vi "bind text.vi"(8 "error in (no error)":errorcluster, 10 "String":string, 11 "SQLite3LV Cursor in":refnum<class "cursor.lvclass">) -> (0 "error out":errorcluster, 3 "SQLite3LV Cursor out":refnum<class "cursor.lvclass">)   [LabVIEW 2014, in "SQLite3LV.lvlib" / "cursor.lvclass"]
uses:
  cursor.lvclass
  cursor.lvclass/cursor.ctl
  SQLite3LV.lvlib
  sqlite3_64.dll
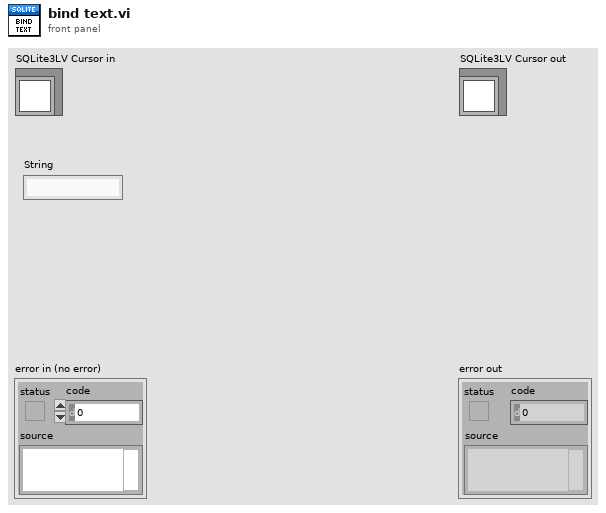
[diagram p1: front panel]
types:
  T1 = typedef "SQLite3LV.lvlib/cursor.lvclass/ctl_active_statement.ctl" = cluster{"ppStmt":i64, "column count":i32, "bind offset":i32, "bind param count":i32, "finished?":bool, "column offset":i32, "column types":i32[]}
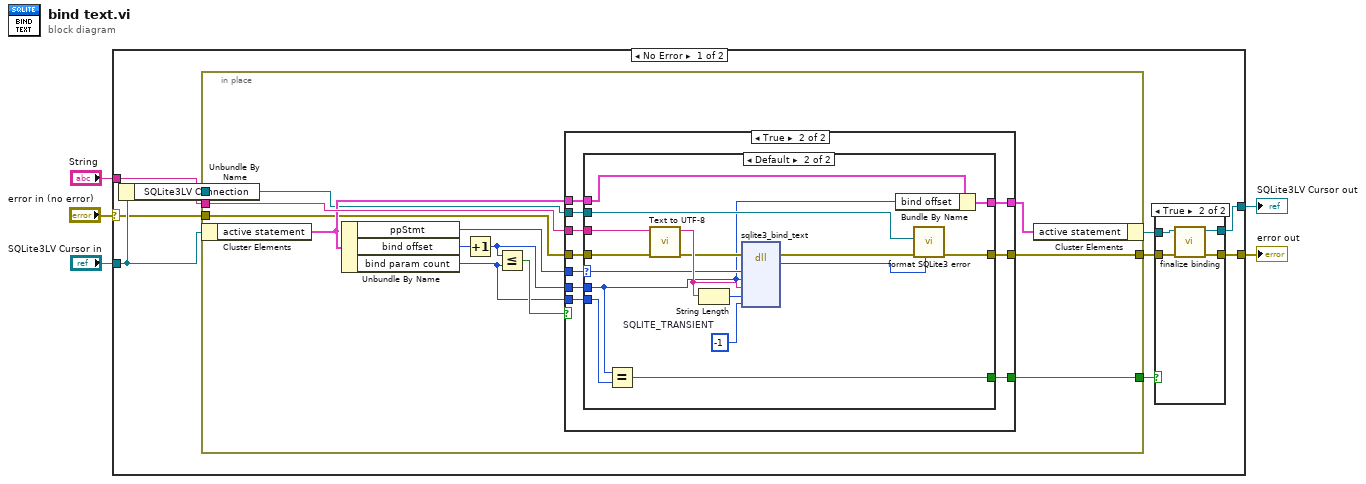
[diagram p0: block diagram]
diagram:
  n1 = case shown="No Error" "error in (no error)" {
    selector: "error in (no error)" -> [w7 w63]
    tunnel: [w10 w63] -> w4
    tunnel: [w12 w62] -> w3
    tunnel: "SQLite3LV Cursor in" -> [w9 w62]
    tunnel: "String" -> [w14 _]
    frame No Error {
      n2 = Unbundle By Name(w9) -> ("SQLite3LV Connection"=w8:refnum<class "sqlite3.lvclass">)
      n3 = in-place {
        in-place-border: w14 -> [w32]
        in-place-border: [w31] -> w11
        in-place-border: w8 -> [w24]
        in-place-border: w7 -> [w23]
        in-place-border: [w21] -> w6
        n4 = in-place-cluster #1(w9) -> ("active statement"=w26:T1)
        n5 = Unbundle By Name(w26) -> ("ppStmt"=w30:i64, "bind offset"=w29:i32, "bind param count"=w22:i32)
        n6 = Increment(x=w29) -> (x+1=w28:i32)
        n7 = Less Or Equal?(x=w28, y=w22) -> (x <= y?=w27:bool)
        n8 = case shown="True" w27 {
          tunnel: w26 -> [w33 w43]
          tunnel: w32 -> [_ w40]
          tunnel: [w33 w42] -> w25
          tunnel: [_ w41] -> w31
          tunnel: w30 -> [_ w37]
          tunnel: w28 -> [_ w39]
          tunnel: w24 -> [_ w38]
          tunnel: w23 -> [_ w36]
          tunnel: w22 -> [_ w35]
          tunnel: [_ w34] -> w21
          frame False {
          }
          frame True {
            n9 = case shown="Default" w37 {
              selector: w37 -> [_ w50]
              tunnel: w43 -> [w44 w61]
              tunnel: [w44 w60] -> w42
              tunnel: [w45 w59] -> w41
              tunnel: w40 -> [_ w58]
              tunnel: w39 -> [_ w48]
              tunnel: w38 -> [_ w57]
              tunnel: w36 -> [w45 w49]
              tunnel: w35 -> [_ w47]
              tunnel: [_ w46] -> w34
              frame 0 {
              }
              frame Default {
                w56 = i64 -1  # SQLITE_TRANSIENT
                n10 = Equal?(x=w48, y=w47) -> (x = y?=w46:bool)
                n11 = call "Text to UTF-8.vi"("error in"=w49, "text"=w58) -> ("error out"=w51:errorcluster, "utf-8 text"=w52:string)  [unwired: 8 in]
                n12 = String Length(string=w52) -> (length=w55:i32)
                n13 = dll-call lib="C:/Users/BobUser/Desktop/LVTables/sqlite3**.*" fn="sqlite3_bind_text"(error in=w51, "pStmt"=w50, "index"=w48, "value"=w52, "nBytes"=w55, "pDestruct_NULL"=w56) -> (error out=w53:errorcluster, "column count"=w54:i32)  [unwired: 7 in, 1 out]
                n14 = Bundle By Name(cluster=w61, "bind offset"=w48) -> (w60:T1)
                n15 = call "format SQLite3 error.vi"("SQLite3LV Connection result"=w54, "error in (no error)"=w53, "psqlite"=w57) -> ("error out"=w59:errorcluster)  [unwired: 8 in]
              }
            }
          }
        }
        n16 = in-place-cluster #1("active statement"=w25) -> (w13:refnum<class "cursor.lvclass">)
      }
      n17 = case shown="True" w6 {
        tunnel: w13 -> [w16 w20]
        tunnel: [w16 w19] -> w12
        tunnel: w11 -> [w15 w18]
        tunnel: [w15 w17] -> w10
        frame False {
        }
        frame True {
          n18 = call "finalize binding.vi"("error in (no error)"=w18, "SQLite3LV Cursor in"=w20) -> ("error out"=w17:errorcluster, "SQLite3LV Cursor out"=w19:refnum<class "cursor.lvclass">)  [unwired: 8 in]
        }
      }
    }
    frame Error {
    }
  }
  "error out" <- w4
  "SQLite3LV Cursor out" <- w3
